vi "BSP.vi"() -> (16 "핀이 남았다":bool)   [LabVIEW 2014]
doc: "The myRIO Project template acquires acceleration data from the onboard accelerometer and displays the changes of acceleration values in a waveform chart."
uses:
  <vilib>/vision/driver/NI_Vision_Acquisition_Software.lvlib
  <vilib>/vision/NI_Vision_Development_Module.lvlib
panel:
  in  "몇초뒤 정지":u32=1000
  in  "Threshold Color Mode 3":enum32{"RGB", "HSL"}(radio)=enum."HSL"
  out "볼링핀이 있는가?":bool=TRUE
  in  "화면전환":bool=TRUE
  out "Image 3":T1(plugin-control)
  in  "탭컨트롤":dbl
  in  "탭 컨트롤":enum32{"볼링핀 0", "녹색핀 1"}(tab)
  in  "Blue or Luminance 3":cluster{i32, i32}(slide)={60, 255} scale=0.0..255.0
  in  "Green or Saturation 3":cluster{i32, i32}(slide)={35, 255} scale=0.0..255.0
  in  "Red or Hue 3":cluster{i32, i32}(slide)={50, 130} scale=0.0..255.0
  in  "Number of Erosion":i32=2
  in  "Threshold Color Mode":enum32{"RGB", "HSL"}(radio)=enum."HSL"
  out "Image 2":T1(plugin-control)
  out "Image":T1(plugin-control)
  in  "Camera Name":refnum<k21>="cam1" caption="IMAQdx Session"
  # "Control Motor"
  # "Read Encoder"
  # "배경색(검은색) 색조"
  # "HSL : 색조 채도 광도"
  # "흰색 : 0/255"
  # "흰색 : 0~55"
  # "흰색 : 135~255"
  # "녹색 : 50/130"
  # "녹색 : 35/255"
  # "녹색 : 60/255"
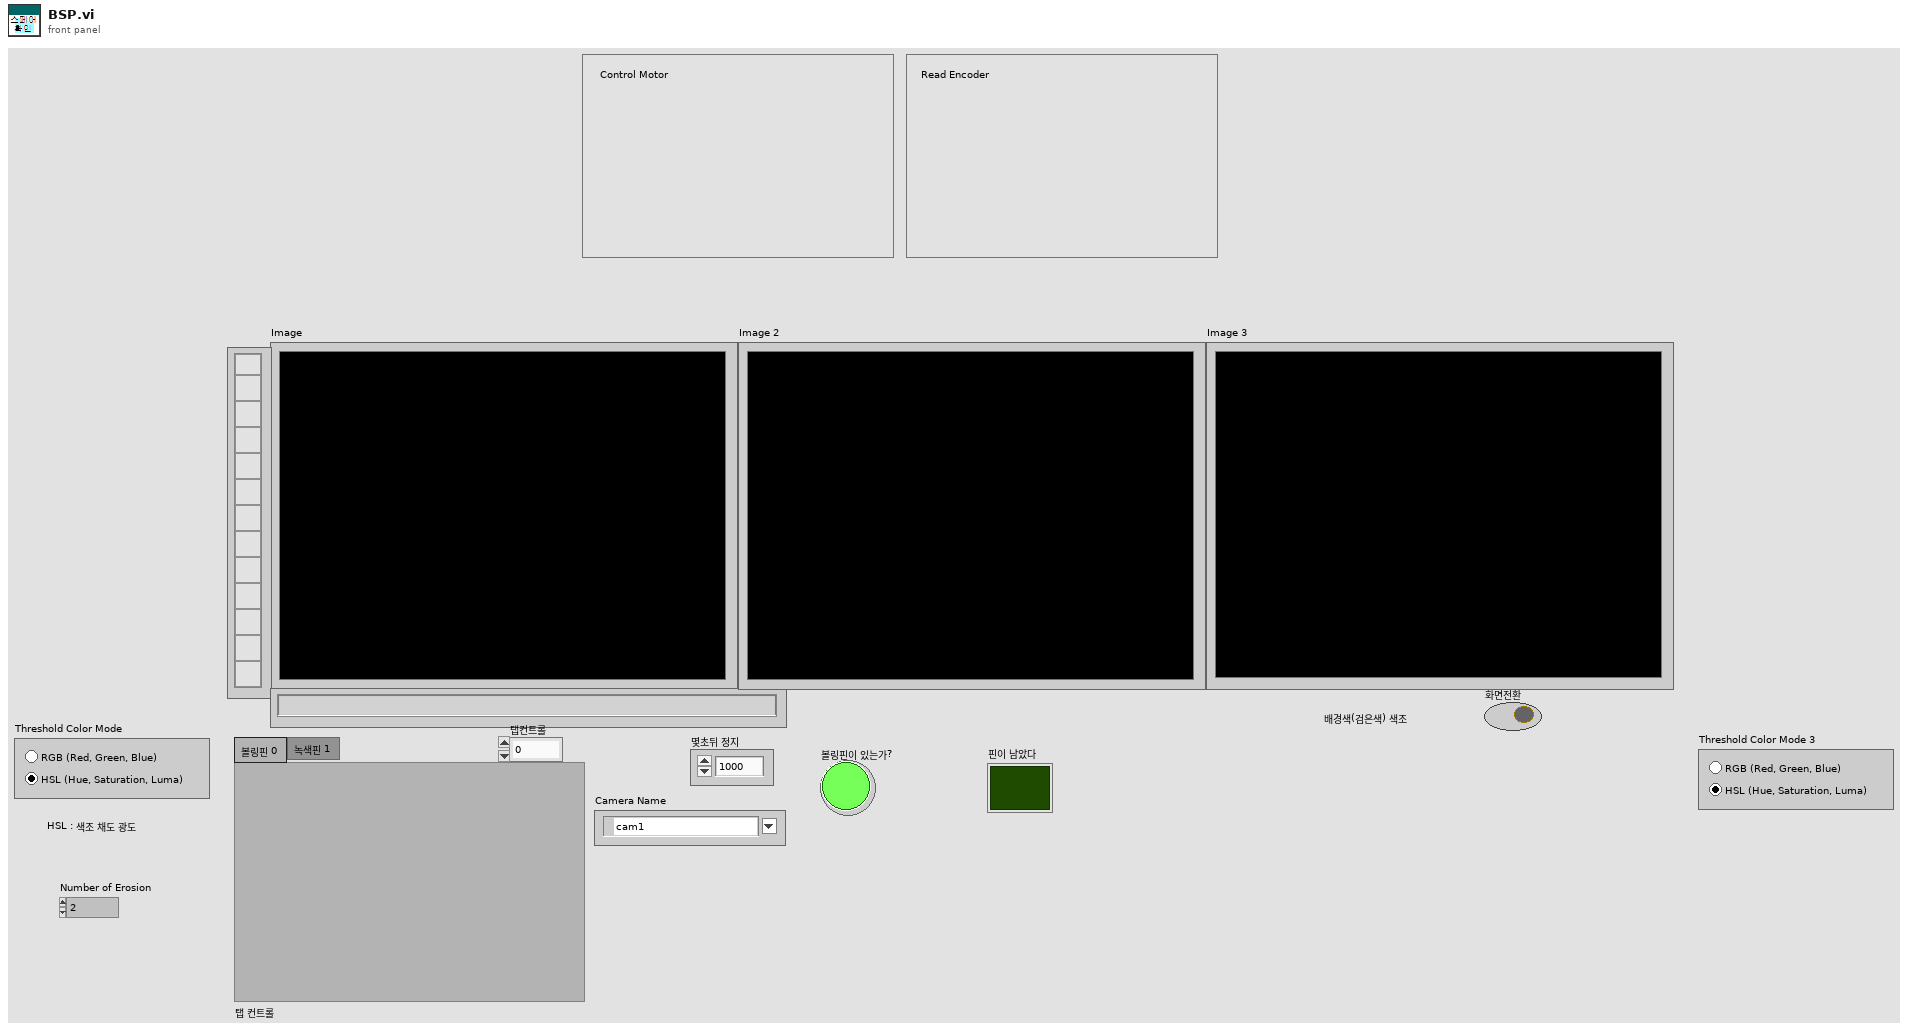
[diagram p1: front panel]
types:
  T1 = typedef "IMAQ Image.ctl" = refnum<image>
  T2 = typedef "IMAQ Rectangle" = cluster{"Left":i32, "Top":i32, "Right":i32, "Bottom":i32, "Rotation":dbl}
  T3 = typedef "Image Type" = u32
  T4 = typedef "IMAQdx.ctl" = refnum<k21>
  T5 = cluster{"Area":dbl, "Number of Holes":dbl, "Bounding Rect":cluster{"Left":dbl, "Top":dbl, "Right":dbl, "Bottom":dbl}, "Center of Mass":cluster{"X":dbl, "Y":dbl}, "Orientation":dbl, "Dimensions":cluster{"Width":dbl, "Height":dbl}}[]
  T6 = cluster{"Area":dbl, "Number of Holes":dbl, "Bounding Rect":cluster{"Left":dbl, "Top":dbl, "Right":dbl, "Bottom":dbl}, "Center of Mass":cluster{"X":dbl, "Y":dbl}, "Orientation":dbl, "Dimensions":cluster{"Width":dbl, "Height":dbl}}
  T7 = cluster{"Left":dbl, "Top":dbl, "Right":dbl, "Bottom":dbl}
  T8 = typedef "ROI Descriptor" = cluster{"Global Rectangle":i32[], "Contours":cluster{"ID":enum32{"External", "Internal"}, "Type":u32, "Coordinates":i32[]}[]}
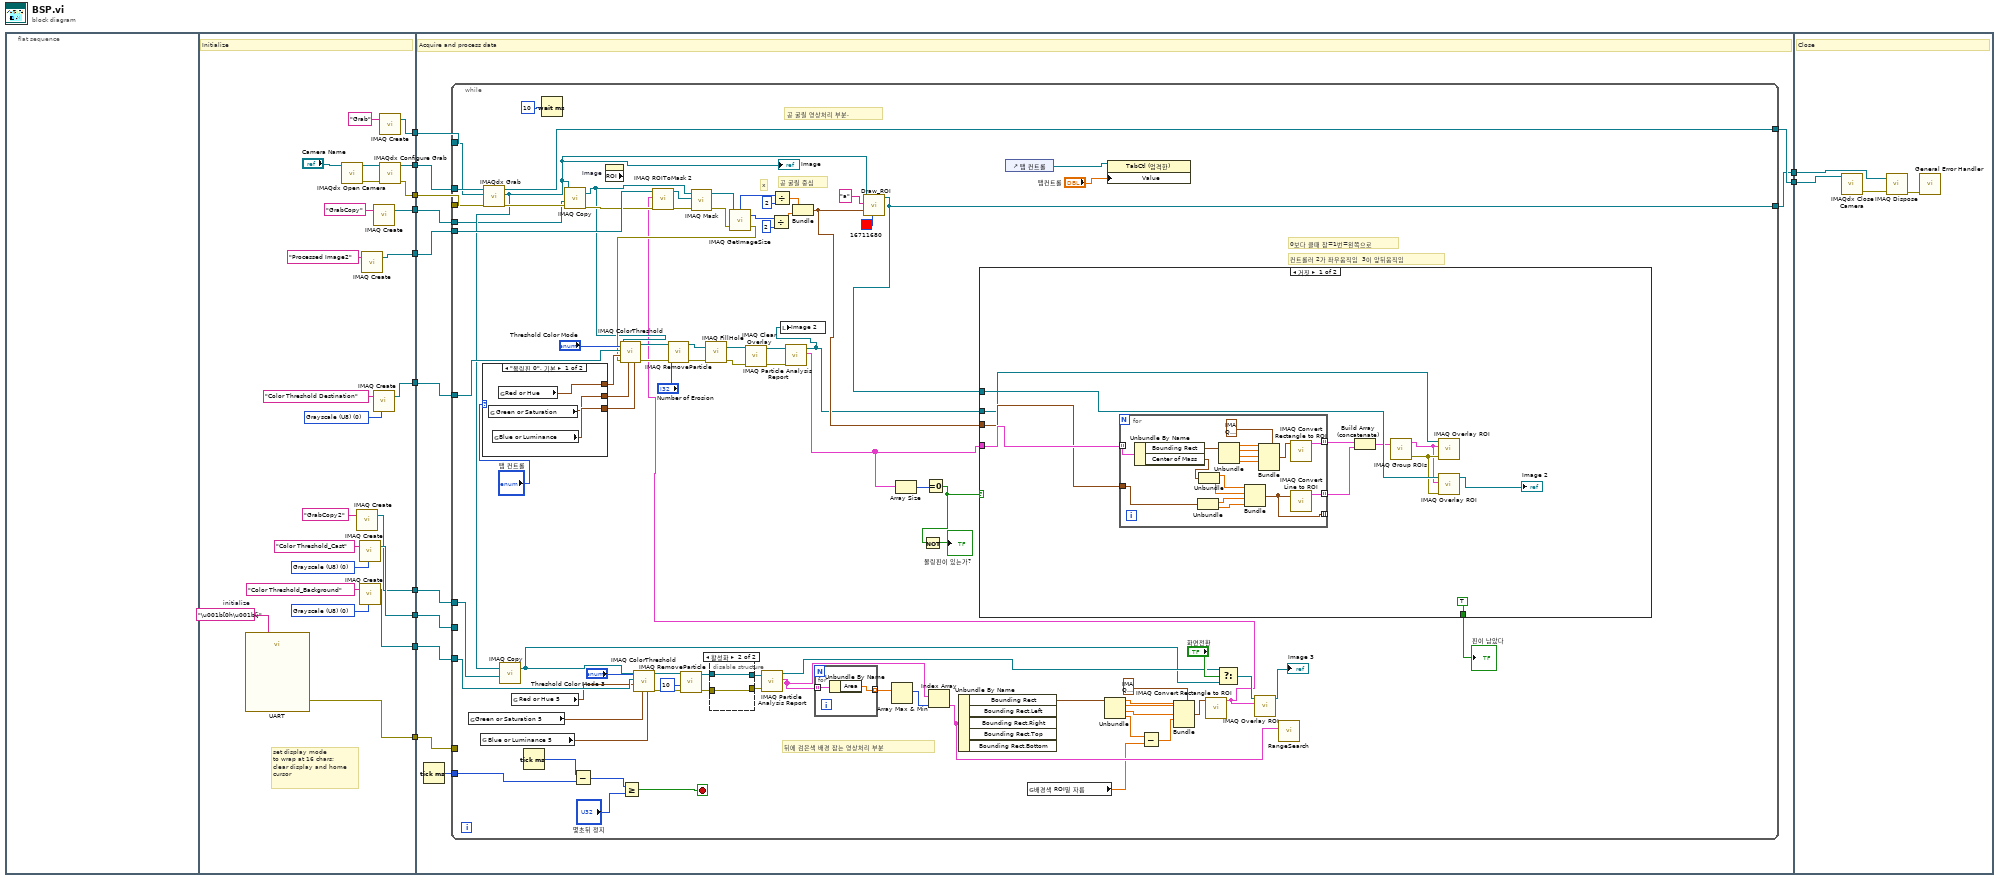
[diagram p0: block diagram]
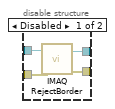
[diagram p2: hidden frame]
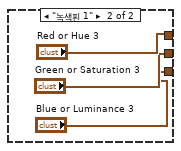
[diagram p3: hidden frame]
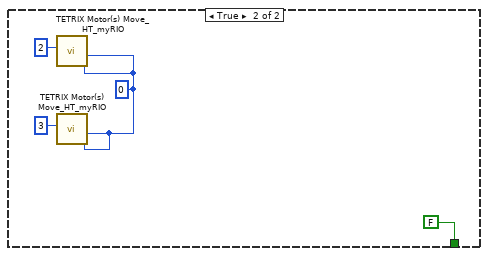
[diagram p4: hidden frame]
diagram:
  n1 = flat-sequence {
    tunnel: [w32] -> w12
    tunnel: [w31] -> w11
    tunnel: [w30] -> w10
    tunnel: [w28] -> w9
    tunnel: [w26] -> w8
    tunnel: [w25] -> w7
    tunnel: [w22] -> w6
    tunnel: [w18] -> w5
    tunnel: [w15] -> w4
    tunnel: [w13] -> w3
    tunnel: w12 -> [w49]
    tunnel: w11 -> [w48]
    tunnel: w10 -> [w47]
    tunnel: [w43] -> w2
    tunnel: [w46] -> w1
    tunnel: w9 -> [w45]
    tunnel: w8 -> [w44]
    tunnel: w7 -> [w38]
    tunnel: w6 -> [w42]
    tunnel: w5 -> [w41]
    tunnel: w4 -> [w40]
    tunnel: w3 -> [w39]
    tunnel: w2 -> [w183]
    tunnel: w1 -> [w182]
    frame #0 {
    }
    frame #1 {
      w16 = T3 0 items=["Grayscale (U8)", "Grayscale (I16)", "Grayscale (SGL)", "Complex (CSG)", "RGB (U32)", "HSL (U32)", "RGB (U64)", "Grayscale (U16)"] ("Image Type")
      w19 = T3 0 items=["Grayscale (U8)", "Grayscale (I16)", "Grayscale (SGL)", "Complex (CSG)", "RGB (U32)", "HSL (U32)", "RGB (U64)", "Grayscale (U16)"] ("Image Type")
      w21 = "\u001b[0h\u001b[j"  # initialize
      w24 = T3 0 items=["Grayscale (U8)", "Grayscale (I16)", "Grayscale (SGL)", "Complex (CSG)", "RGB (U32)", "HSL (U32)", "RGB (U64)", "Grayscale (U16)"] ("Image Type")
      # "set display mode\nto wrap at 16 chars;\nclear display and home\ncursor"
      # "Initialize"
      n2 = call "UART"("Characters to Write"=w21) -> ("error out"=w25:errorcluster)  [unwired: 25 in, 1 out]
      n3 = call <vilib>:"IMAQdx Open Camera.vi"("Session In"="Camera Name") -> ("error out"=w36:errorcluster, "Session Out"=w35:T4)  [unwired: 2 in, 7 out]
      n4 = call "IMAQ Create"("Image Name"="GrabCopy2") -> ("New Image"=w13:T1)  [unwired: 3 in, 2 out]
      n5 = call "IMAQ Create"("Image Name"="Color Threshold_Cast", "Image Type"=w16) -> ("New Image"=w15:T1)  [unwired: 3 in, 1 out]
      n6 = call "IMAQ Create"("Image Name"="Color Threshold_Background", "Image Type"=w19) -> ("New Image"=w18:T1)  [unwired: 3 in, 1 out]
      n7 = call "IMAQ Create"("Image Name"="Processed Image2") -> ("New Image"=w28:T1)  [unwired: 3 in, 2 out]
      n8 = call "IMAQ Create"("Image Name"="Color Threshold Destination", "Image Type"=w24) -> ("New Image"=w22:T1)  [unwired: 3 in, 1 out]
      n9 = call "IMAQ Create"("Image Name"="GrabCopy") -> ("New Image"=w26:T1)  [unwired: 3 in, 2 out]
      n10 = call "IMAQ Create"("Image Name"="Grab") -> ("New Image"=w32:T1)  [unwired: 3 in, 2 out]
      n11 = call <vilib>:"IMAQdx Configure Grab.vi"("error in"=w36, "Session In"=w35) -> ("error out"=w30:errorcluster, "Session Out"=w31:T4)  [unwired: 8 out]
    }
    frame #2 {
      # "Acquire and process data"
      n12 = Tick Count (ms)() -> (millisecond timer value=w37:u32)
      n13 = while {
        tunnel: [w132] -> w46
        tunnel: w47 -> [w134]
        tunnel: w48 -> [w135]
        tunnel: w49 -> [w133]
        tunnel: w45 -> [w130]
        tunnel: w44 -> [w65]
        tunnel: [w99] -> w43
        tunnel: w38 -> [_]
        tunnel: w42 -> [w117]
        tunnel: w41 -> [w75]
        tunnel: w40 -> [_]
        tunnel: w39 -> [w91]
        tunnel: w37 -> [w57]
        stop <- w55 stop-if-true
        # "뒤에 검은색 배경 잡는 영상처리 부분"
        # "공 굴릴 영상처리 부분."
        # "0보다 클때 참=1번=왼쪽으로"
        # "컨트롤러 2가 좌우움직임  3이 앞뒤움직임"
        # "공 굴릴 중심"
        # "x"
        n14 = global read "글로벌.vi" "Green or Saturation 5"() -> (w52:cluster{i32, i32})
        n15 = global read "글로벌.vi" "Blue or Luminance 5"() -> (w50:cluster{i32, i32})
        n16 = case shown="\"볼링핀 0\", 기본" "탭 컨트롤" {
          tunnel: [w146 "Blue or Luminance 3"] -> w115
          tunnel: [w144 "Red or Hue 3"] -> w114
          tunnel: [w145 "Green or Saturation 3"] -> w113
          frame "볼링핀 0", Default {
            n17 = global read "글로벌.vi" "Green or Saturation"() -> (w145:cluster{i32, i32})
            n18 = global read "글로벌.vi" "Blue or Luminance"() -> (w146:cluster{i32, i32})
            n19 = global read "글로벌.vi" "Red or Hue"() -> (w144:cluster{i32, i32})
          }
          frame "녹색핀 1" {
          }
        }
        n20 = call <vilib>:"IMAQdx Grab.vi"("error in"=w134, "Image In"=w133, "Session In"=w135) -> ("error out"=w120:errorcluster, "Image Out"=w66:T1, "Session Out"=w132:T4)  [unwired: 1 in, 5 out]
        "Image" <- w66
        n21 = call "IMAQ Copy"("Image Dst"=w91, "Image Src"=w66) -> ("Image Dst Out"=w71:T1)  [unwired: 4 in, 1 out]
        n22 = global read "글로벌.vi" "Red or Hue 5"() -> (w51:cluster{i32, i32})
        n23 = Tick Count (ms)() -> (millisecond timer value=w58:u32)
        n24 = Wait (ms)(milliseconds to wait=u32 10 ("대기 시간(ms)")) -> ()  [unwired: 1 out]
        n25 = call "IMAQ Copy"("error in (no error)"=w120, "Image Dst"=w65, "Image Src"=w66) -> ("error out"=w119:errorcluster, "Image Dst Out"=w63:T1)  [unwired: 3 in]
        n26 = Subtract(x=w58, y=w57) -> (x-y=w56:u32)
        n27 = property on="Image" class="ImageControl" props=["ROI"]() -> ()  [unwired: 2 in, 3 out]
        n28 = Greater Or Equal?(x=w56, y="몇초뒤 정지") -> (x >= y?=w55:bool)
        n29 = call "IMAQ ColorThreshold"("Blue or Luma or Val or Inten Range"=w50, "Green or Sat Range"=w52, "Color Mode"="Threshold Color Mode 3", "Red or Hue Range"=w51, "Image Dst"=w75, "Image Src"=w71) -> ("error out"=w80:errorcluster, "Image Dst Out"=w79:T1)  [unwired: 4 in]
        n30 = call "IMAQ RemoveParticle"("error in (no error)"=w80, "Number of Erosion"=10, "Image Src"=w79) -> ("error out"=w82:errorcluster, "Image Dst Out"=w81:T1)  [unwired: 7 in]
        n31 = disable-structure shown="활성화" {
          disable-tunnel: w81 -> [w139 w141]
          disable-tunnel: w82 -> [w138 w140]
          disable-tunnel: [w137 w141] -> w84
          disable-tunnel: [w136 w140] -> w85
          frame Disabled {
            n32 = call "IMAQ RejectBorder"("error in (no error)"=w138, "Image Src"=w139) -> ("error out"=w136:errorcluster, "Image Dst Out"=w137:T1)  [unwired: 4 in]
          }
          frame Enabled {
          }
        }
        n33 = call "IMAQ Particle Analysis Report"("error in (no error)"=w85, "Image"=w84) -> ("Particle Reports (Pixels)"=w77:T5, "Image Out (duplicate)"=w76:T1)  [unwired: 4 in, 4 out]
        n34 = for {
          tunnel: w77 -> [w143] mode=indexing
          tunnel: [w142] -> w97 mode=indexing
          n35 = Unbundle By Name(w143) -> ("Area"=w142:dbl)
        }
        n36 = Array Max & Min(array=w97) -> (max index (indices)=w96:i32)  [unwired: 3 out]
        n37 = Index Array(array=w77, index=w96) -> (element=w89:T6)
        n38 = Unbundle By Name(w89) -> ("Bounding Rect"=w93:T7)  [unwired: 4 out]
        n39 = control-ref of="탭 컨트롤"() -> (w103:refnum<vi>)
        n40 = global read "글로벌.vi" "배경색 ROI밑 자름"() -> (w53:dbl)
        n41 = Unbundle(w93) -> ("Left"=w74:dbl, "Top"=w94:dbl, "Right"=w73:dbl, "Bottom"=w70:dbl)
        n42 = property class="TabCtl (엄격한)"(reference=w103, "Value"="탭컨트롤") -> ()  [unwired: 1 in, 2 out]
        n43 = Subtract(x=w70, y=w53) -> (x-y=w69:dbl)
        n44 = Bundle(cluster=T2 {"Left"=0, "Top"=0, "Right"=0, "Bottom"=0, "Rotation"=0.0} ("Rectangle"), "Left"=w74, "Top"=w94, "Right"=w73, "Bottom"=w69) -> (w95:T2)  [unwired: 1 in]
        n45 = call "IMAQ Convert Rectangle to ROI"("Rectangle"=w95) -> ("ROI Descriptor"=w60:T8)  [unwired: 8 in, 1 out]
        n46 = call "IMAQ ROIToMask 2"("error in (no error)"=w119, "ROI Descriptor"=w60, "Image"=w130) -> ("error out"=w129:errorcluster, "Image Out"=w64:T1)  [unwired: 6 in, 1 out]
        n47 = call "IMAQ Mask"("error in (no error)"=w129, "Image Mask"=w64, "Image Src"=w63) -> ("error out"=w118:errorcluster, "Image Dst Out"=w67:T1)  [unwired: 2 in]
        n48 = call "IMAQ GetImageSize"("Image"=w67, "error in (no error)"=w118) -> ("Y Resolution"=w124:i32, "X Resolution"=w127:i32, "error out"=w110:errorcluster)  [unwired: 2 in]
        n49 = call "IMAQ ColorThreshold"("Blue or Luma or Val or Inten Range"=w115, "Green or Sat Range"=w113, "Color Mode"="Threshold Color Mode", "error in (no error)"=w110, "Red or Hue Range"=w114, "Image Dst"=w117, "Image Src"=w63) -> ("error out"=w111:errorcluster, "Image Dst Out"=w72:T1)  [unwired: 3 in]
        n50 = call "IMAQ RemoveParticle"("error in (no error)"=w111, "Number of Erosion"="Number of Erosion", "Image Src"=w72) -> ("error out"=w106:errorcluster, "Image Dst Out"=w107:T1)  [unwired: 7 in]
        n51 = call "IMAQ FillHole"("error in (no error)"=w106, "Image Src"=w107) -> ("error out"=w109:errorcluster, "Image Dst Out"=w108:T1)  [unwired: 4 in]
        n52 = call "IMAQ Clear Overlay"("error in (no error)"=w109, "Image"=w108) -> ("error out"=w128:errorcluster, "Image Out"=w131:T1)  [unwired: 1 in, 7 out]
        n53 = Divide(x=w124, y=2) -> (x/y=w123:dbl)
        n54 = Divide(x=w127, y=2) -> (x/y=w86:dbl)
        n55 = call "IMAQ Particle Analysis Report"("error in (no error)"=w128, "Image"=w131) -> ("Particle Reports (Pixels)"=w68:T5, "Image Out (duplicate)"=w98:T1)  [unwired: 4 in, 4 out]
        n56 = local write "Image 2"(w98) -> ()
        n57 = Bundle(w86, w123) -> (w101:cluster{dbl, dbl})  [unwired: 1 in]
        n58 = call "Draw_ROI.vi"("Color"=u32 16711680, "클러스터"=w101, "Group"="a", "참조 번호 입력"=w66) -> ("참조 번호 출력"=w99:T1)  [unwired: 7 in]
        n59 = Array Size(array=w68) -> (size(s)=w105:i32)
        n60 = Equal To 0?(x=w105) -> (x = 0?=w87:bool)
        n61 = Not(x=w87) -> (.not. x?=→"볼링핀이 있는가?":bool)
        n62 = case shown="거짓" w87 {
          tunnel: w68 -> [w160 _]
          tunnel: w101 -> [w159 _]
          tunnel: w98 -> [w158 _]
          tunnel: w99 -> [w157 _]
          tunnel: [TRUE ("핀이 남았다") FALSE ("핀이 남았다")] -> w59
          frame False {
            n63 = for {
              tunnel: w160 -> [w177] mode=indexing
              tunnel: [w169] -> w153 mode=indexing
              tunnel: w159 -> [w165]
              tunnel: [w162] -> w155 mode=indexing
              tunnel: [w161] -> _ mode=indexing
              n64 = Unbundle By Name(w177) -> ("Bounding Rect"=w175:T7, "Center of Mass"=w168:cluster{"X":dbl, "Y":dbl})
              n65 = Unbundle(w165) -> (w164:dbl, w163:dbl)
              n66 = Unbundle(w168) -> ("X"=w167:dbl, "Y"=w166:dbl)
              n67 = Unbundle(w175) -> ("Left"=w174:dbl, "Top"=w173:dbl, "Right"=w172:dbl, "Bottom"=w171:dbl)
              n68 = Bundle("X"=w167, "Y"=w166, w164, w163) -> (w161:cluster{"X":dbl, "Y":dbl, dbl, dbl})  [unwired: 1 in]
              n69 = Bundle(cluster=T2 {"Left"=0, "Top"=0, "Right"=0, "Bottom"=0, "Rotation"=0.0} ("Rectangle"), "Left"=w174, "Top"=w173, "Right"=w172, "Bottom"=w171) -> (w170:T2)  [unwired: 1 in]
              n70 = call "IMAQ Convert Rectangle to ROI"("Rectangle"=w170) -> ("ROI Descriptor"=w169:T8)  [unwired: 8 in, 1 out]
              n71 = call "IMAQ Convert Line to ROI"("Line"=w161) -> ("ROI Descriptor"=w162:T8)  [unwired: 8 in, 1 out]
            }
            n72 = Build Array (concatenate)(w153, w155) -> (w154:T8[])
            n73 = call "IMAQ Group ROIs"("ROI Descriptors"=w154) -> ("error out"=w156:errorcluster, "ROI Descriptor out"=w152:T8)  [unwired: 1 in, 2 out]
            n74 = call "IMAQ Overlay ROI"("error in (no error)"=w156, "ROI Descriptor"=w152, "Image"=w157) -> ()  [unwired: 3 in, 6 out]
            n75 = call "IMAQ Overlay ROI"("error in (no error)"=w156, "ROI Descriptor"=w152, "Image"=w158) -> ("Image Out"=→"Image 2":T1)  [unwired: 3 in, 5 out]
          }
          frame True {
            w179 = 0
            n76 = call <vilib>:"TETRIX Motor(s) Move_HT_myRIO.vi"("Motor 2 Power (-100 to 100)\n0 = Stop/Brake\n-128 = Stop/Coast"=w179, "Motor 1 Power (-100 to 100)\n0 = Stop/Brake\n-128 = Stop/Coast"=w179, "Controller Daisy Chain Position: 1 - 4"=u8 2) -> ()  [unwired: 6 in, 1 out]
            n77 = call <vilib>:"TETRIX Motor(s) Move_HT_myRIO.vi"("Motor 2 Power (-100 to 100)\n0 = Stop/Brake\n-128 = Stop/Coast"=w179, "Motor 1 Power (-100 to 100)\n0 = Stop/Brake\n-128 = Stop/Coast"=w179, "Controller Daisy Chain Position: 1 - 4"=u8 3) -> ()  [unwired: 6 in, 1 out]
          }
        }
        "핀이 남았다" <- w59
        n78 = Select(t=w76, s="화면전환", f=w71) -> (s? t:f=w62:T1)
        n79 = call "IMAQ Overlay ROI"("ROI Descriptor"=w60, "Image"=w62) -> ("Image Out"=→"Image 3":T1)  [unwired: 4 in, 5 out]
        n80 = call "RangeSearch.vi"("Particle Report"=w89) -> ()  [unwired: 10 in, 1 out]
      }
    }
    frame #3 {
      # "Close"
      n81 = call <vilib>:"IMAQdx Close Camera.vi"("Session In"=w182) -> ("error out"=w185:errorcluster)  [unwired: 1 in, 9 out]
      n82 = call "IMAQ Dispose"("Image"=w183, "error in (no error)"=w185) -> ("error out"=w184:errorcluster)  [unwired: 4 in]
      n83 = call <vilib>:"General Error Handler.vi"("error in (no error)"=w184) -> ()  [unwired: 2 in, 13 out]
    }
  }
